vi "Get Plugin Components.vi"(8 "error in (no error)":errorcluster, 11 "Item Ref in":T1 format="%.0x") -> (0 "error out":errorcluster, 2 "Plugin Components":refnum<class "Component.lvclass">[](array[class]), 3 "Item Ref out":T1 format="%.0x")   [LabVIEW 2017, in "DSF System Explorer.lvlib"]
uses:
  DSF System Explorer.lvlib
  <vilib>/NI Veristand/Custom Device API/Custom Device Item Ref.ctl
  DSF Core.lvlibp/Classes/Component/Component.lvclass
  Shared/DSF Shared.lvlib
  <vilib>/NI Veristand/Custom Device API/Custom Device API.lvlib
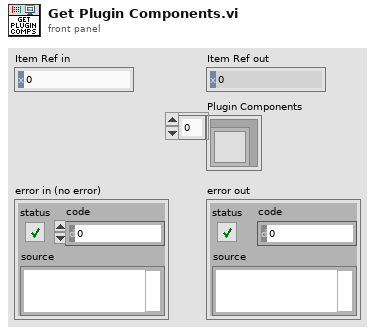
[diagram p1: front panel]
types:
  T1 = typedef "Custom Device API.lvlib/Custom Device Item Ref.ctl" = u64
  T2 = typedef "DSF Core.lvlibp/Plugin Configuration.lvclass/Core Plugin Configuration.ctl" = cluster{"name":string, "components":string[], "cycle timing":T3}
  T3 = typedef "DSF Core.lvlibp/DSF Timing Info.ctl" = cluster{"priority":u64, "decimation":u64, "offset":u64}
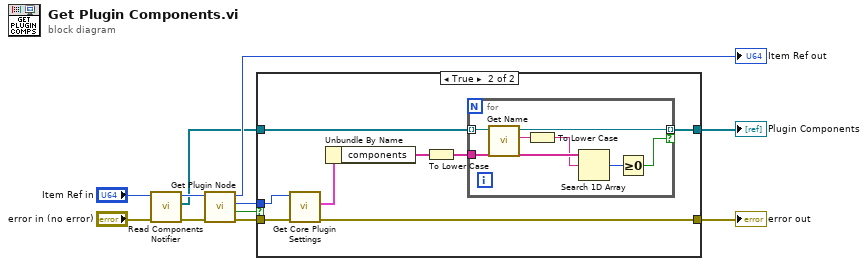
[diagram p0: block diagram]
diagram:
  n1 = call "Read Components Notifier.vi"("error in (no error)"="error in (no error)", "Item Ref in"="Item Ref in") -> ("error out"=w6:errorcluster, "Components"=w3:refnum<class "Component.lvclass">[], "Item Ref out"=w5:T1)  [unwired: 7 in]
  n2 = call "Get Plugin Node.vi"("error in (no error)"=w6, "Item Ref in"=w5) -> ("error out"=w11:errorcluster, "found?"=w10:bool, "Plugin Ref"=w9:T1, "Item Ref out"=→"Item Ref out":T1)  [unwired: 6 in]
  n3 = case shown="True" w10 {
    tunnel: w11 -> [w12 w20]
    tunnel: w9 -> [_ w19]
    tunnel: w3 -> [_ w16]
    tunnel: [_ w15] -> w2
    tunnel: [w12 w14] -> w1
    frame False {
    }
    frame True {
      n4 = call "Get Core Plugin Settings.vi"("error in (no error)"=w20, "Item Ref in"=w19) -> ("error out"=w14:errorcluster, "plugin configuration"=w18:T2)  [unwired: 7 in, 1 out]
      n5 = Unbundle By Name(w18) -> ("components"=w17:string[])
      n6 = To Lower Case(string=w17) -> (all lower case string=w13:string[])
      n7 = for {
        tunnel: w13 -> [w27]
        tunnel: w16 -> [w26] mode=indexing
        tunnel: [w24] -> w15 mode=indexing if=w22
        n8 = call "Get Name.vi"("Component in"=w26) -> ("name"=w25:string, "Component out"=w24:refnum<class "Component.lvclass">)  [unwired: 9 in]
        n9 = To Lower Case(string=w25) -> (all lower case string=w21:string)
        n10 = Search 1D Array(1D array=w27, element=w21) -> (index of element=w23:i32)  [unwired: 1 in]
        n11 = Greater Or Equal To 0?(x=w23) -> (x >= 0?=w22:bool)
      }
    }
  }
  "error out" <- w1
  "Plugin Components" <- w2
